vi "ignoreTimeout.vi"(8 "error in (no error)":errorcluster) -> (0 "error out":errorcluster)   [LabVIEW 2017]
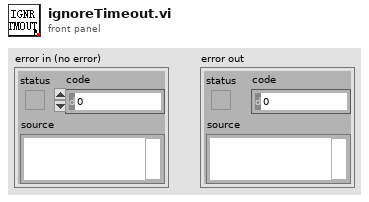
[diagram p1: front panel]
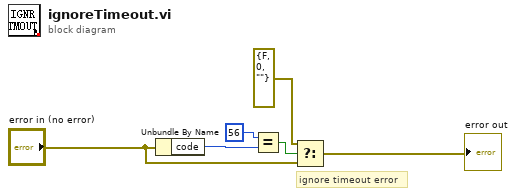
[diagram p0: block diagram]
diagram:
  # "ignore timeout error"
  n1 = Unbundle By Name("error in (no error)") -> ("code"=w1:i32)
  n2 = Equal?(x=56, y=w1) -> (x = y?=w3:bool)
  n3 = Select(t=errorcluster {"status"=FALSE, "code"=0, "source"=""}, s=w3, f="error in (no error)") -> (s? t:f=→"error out":errorcluster)
